vi "LvIRKit_ManageIRData.vi"(7 "filepath":path=path "C:/EISOL/LvIRKIt/samples/sample.dat", 8 "action":T2(ring)=enum."Get", 9 "irdata":string, 10 "name":string, 11 "id":i32) -> (1 "irdata out":T1, 2 "IRDATA[]":T1[](array[typedef]))   [LabVIEW 2014]
uses:
  LvIRKit_rsc_IRData_typedef.ctl
panel:
  out "size of IRDATA[]":i32
  in  "irdata":T1
  # "JSONstring"
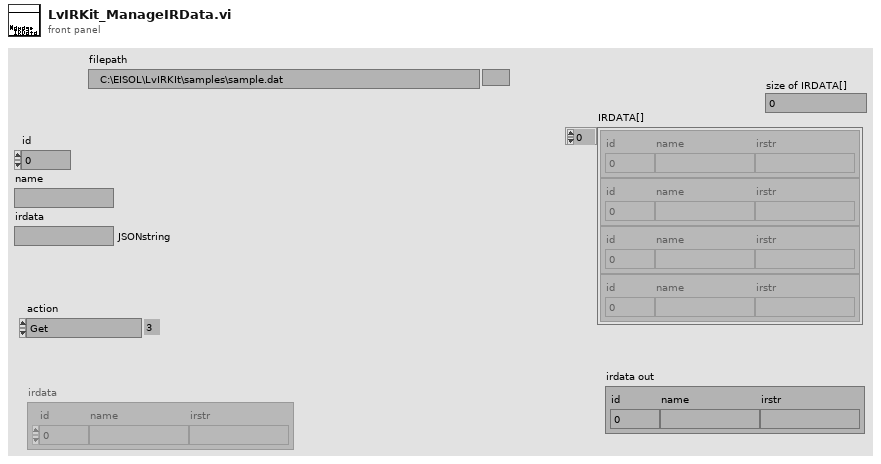
[diagram p1: front panel]
types:
  T1 = typedef "LvIRKit_rsc_IRData_typedef.ctl" = cluster{"id":i32, "name":string, "irstr":string}
  T2 = enum16{"Init", "Load", "Save", "Get", "Add", "Remove", "Replace", "Up", "Down"}
  T3 = enum16{"open", "replace", "create", "open or create", "replace or create", "replace or create with confirmation"}
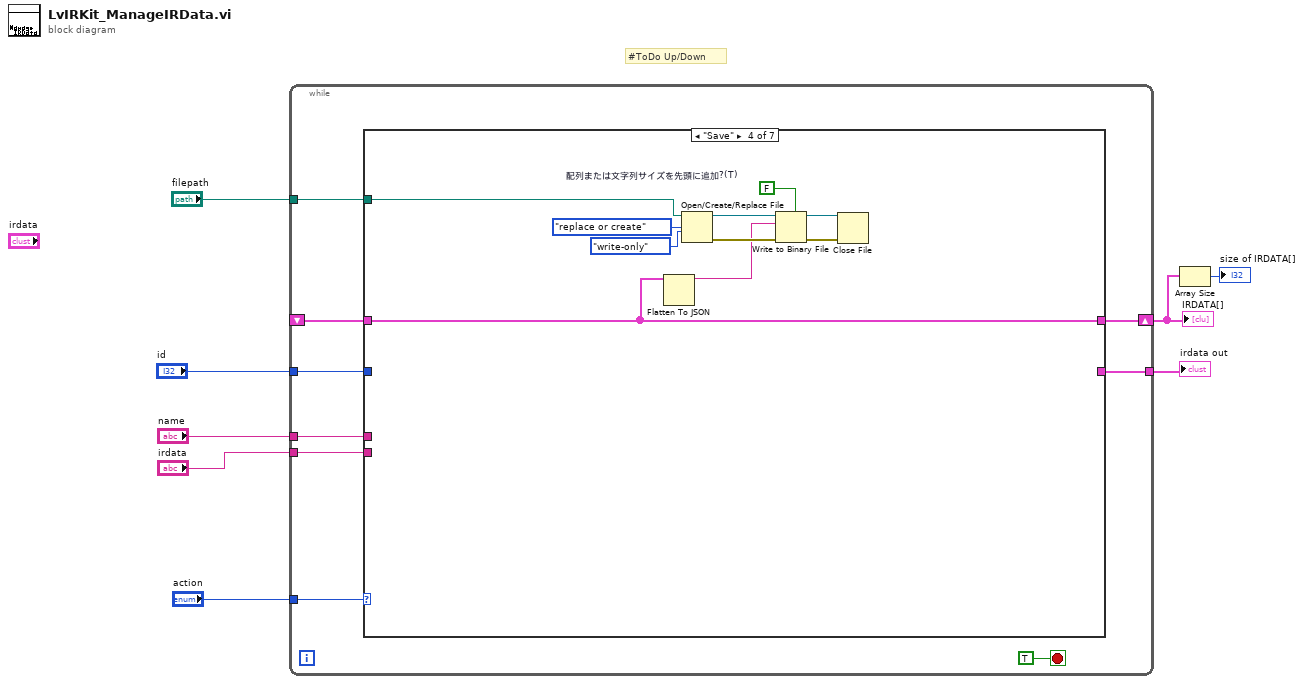
[diagram p0: block diagram]
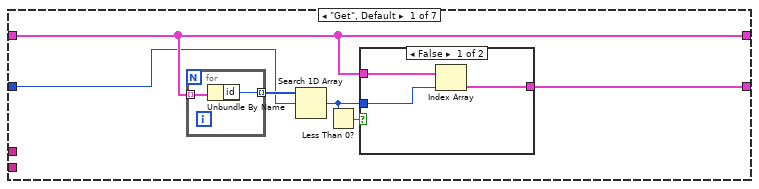
[diagram p2: hidden frame]
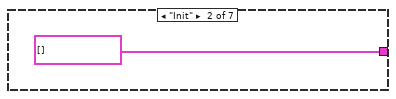
[diagram p4: hidden frame]
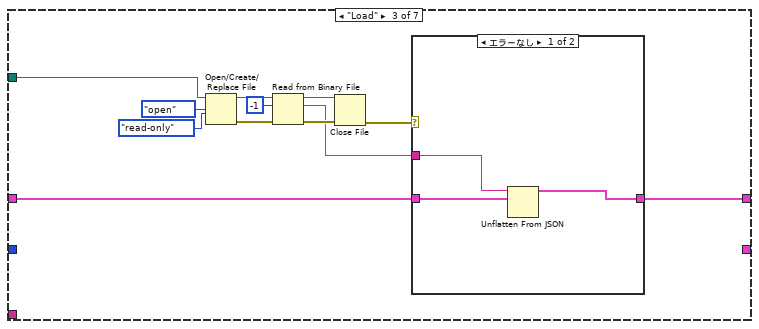
[diagram p5: hidden frame]
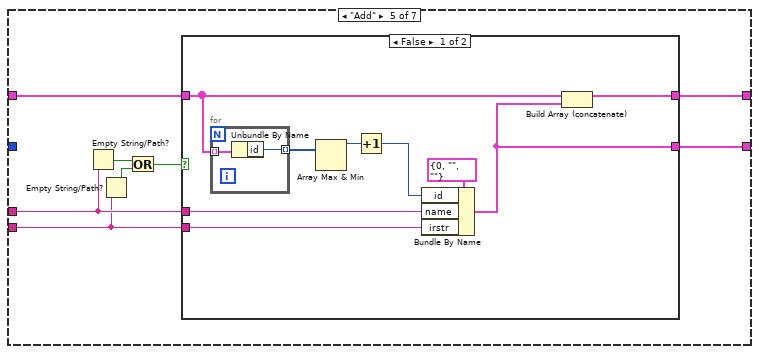
[diagram p7: hidden frame]
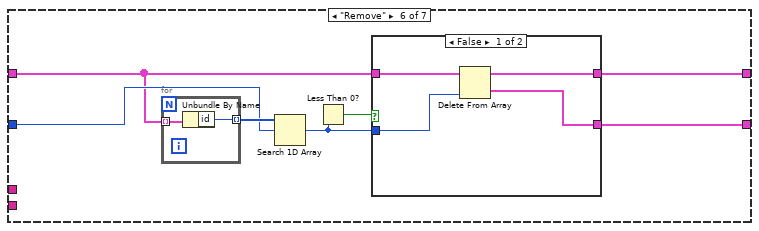
[diagram p9: hidden frame]
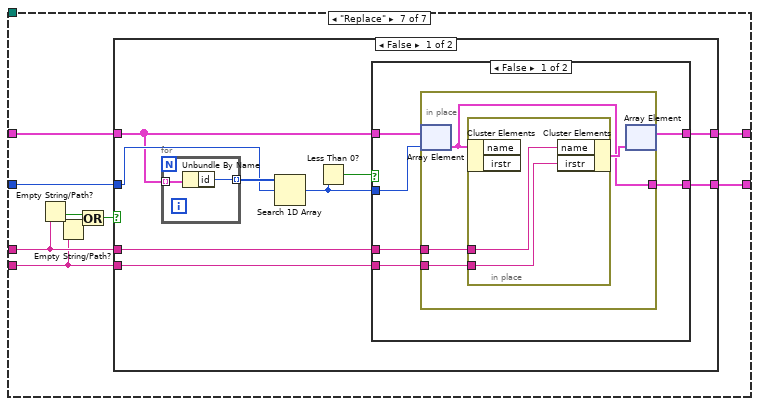
[diagram p11: hidden frame]
diagram:
  # "#ToDo Up/Down"
  n1 = while {
    tunnel: "action" -> [w16]
    shift-right: [w15] -> w2
    shift-left: _ -> [w14]
    tunnel: "id" -> [w13]
    tunnel: [w12] -> w6
    tunnel: "name" -> [w11]
    tunnel: "irdata" -> [w10]
    tunnel: "filepath" -> [w9]
    stop <- TRUE stop-if-true
    n2 = case shown="\"Save\"" w16 {
      tunnel: [w22 T1[] [] ("IRDATA[]") w32 w49 w63 w77 w96] -> w15
      tunnel: w14 -> [w22 _ w33 w49 w62 w78 w97]
      tunnel: w13 -> [w20 _ _ _ _ w81 w98]
      tunnel: [w23 _ _ _ w61 w76 w95] -> w12
      tunnel: w11 -> [_ _ _ _ w60 _ w94]
      tunnel: w10 -> [_ _ _ _ w59 _ w93]
      tunnel: w9 -> [_ _ w31 w46 _ _ _]
      frame "Get", Default {
        n3 = for {
          tunnel: w22 -> [w28] mode=indexing
          tunnel: [w27] -> w21 mode=indexing
          n4 = Unbundle By Name(w28) -> ("id"=w27:i32)
        }
        n5 = Search 1D Array(1D array=w21, element=w20) -> (index of element=w19:i32)  [unwired: 1 in]
        n6 = Less Than 0?(x=w19) -> (x < 0?=w18:bool)
        n7 = case shown="FALSE" w18 {
          tunnel: [w26 _] -> w23
          tunnel: w22 -> [w25 _]
          tunnel: w19 -> [w24 _]
          frame False {
            n8 = Index Array(array=w25, index=w24) -> (element=w26:T1)
          }
          frame True {
          }
        }
      }
      frame "Init" {
      }
      frame "Load" {
        n9 = Open/Create/Replace File(file path (use dialog)=w31, operation (0:open)=T3."open" ("操作（0:open）"), access (0:read/write)=enum16{"read/write", "read-only", "write-only"}."read-only" ("アクセス （0:read/write）")) -> (refnum out=w41:refnum<file>, error out=w40:errorcluster)  [unwired: 3 in, 1 out]
        n10 = Read from Binary File(8:w40, 10:-1 ("カウント（1）"), 11:w41) -> (0:w36:errorcluster, 2:w34:string, 3:w37:refnum<file>)  [unwired: 3 in, 1 out]
        n11 = Close File(refnum=w37, error in=w36) -> (error out=w35:errorcluster)  [unwired: 1 out]
        n12 = case shown="エラーなし" w35 {
          tunnel: w34 -> [w43 _]
          tunnel: w33 -> [w44 w45]
          tunnel: [w42 w45] -> w32
          frame No Error {
            n13 = Unflatten From JSON(JSON string=w43, type and defaults=w44) -> (value=w42:T1[])  [unwired: 5 in, 1 out]
          }
          frame Error {
          }
        }
      }
      frame "Save" {
        w47 = FALSE  # 配列または文字列サイズを先頭に追加?(T)
        n14 = Flatten To JSON(anything=w49) -> (JSON string=w48:string)  [unwired: 2 in, 1 out]
        n15 = Open/Create/Replace File(file path (use dialog)=w46, operation (0:open)=T3."replace or create" ("操作（0:open）"), access (0:read/write)=enum16{"read/write", "read-only", "write-only"}."write-only" ("アクセス （0:read/write）")) -> (refnum out=w55:refnum<file>, error out=w54:errorcluster)  [unwired: 3 in, 1 out]
        n16 = Write to Binary File(file (use dialog)=w55, data=w48, error in=w54, 5:w47) -> (refnum out=w51:refnum<file>, error out=w50:errorcluster)  [unwired: 2 in, 1 out]
        n17 = Close File(refnum=w51, error in=w50) -> ()  [unwired: 2 out]
      }
      frame "Add" {
        n18 = Empty String/Path?(string/path=w60) -> (empty?=w58:bool)
        n19 = Empty String/Path?(string/path=w59) -> (empty?=w57:bool)
        n20 = Or(x=w58, y=w57) -> (x .or. y?=w56:bool)
        n21 = case shown="FALSE" w56 {
          tunnel: [w72 w75] -> w63
          tunnel: w60 -> [w70 _]
          tunnel: w59 -> [w69 _]
          tunnel: w62 -> [w68 w75]
          tunnel: [w64 _] -> w61
          frame False {
            n22 = for {
              tunnel: w68 -> [w74] mode=indexing
              tunnel: [w73] -> w67 mode=indexing
              n23 = Unbundle By Name(w74) -> ("id"=w73:i32)
            }
            n24 = Array Max & Min(array=w67) -> (max value=w66:i32)  [unwired: 3 out]
            n25 = Increment(x=w66) -> (x+1=w65:i32)
            n26 = Bundle By Name(cluster=T1 {"id"=0, "name"="", "irstr"=""} ("irdata"), "id"=w65, "name"=w70, "irstr"=w69) -> (w64:T1)
            n27 = Build Array (concatenate)(w68, w64) -> (w72:T1[])
          }
          frame True {
          }
        }
      }
      frame "Remove" {
        n28 = for {
          tunnel: w78 -> [w84] mode=indexing
          tunnel: [w83] -> w82 mode=indexing
          n29 = Unbundle By Name(w84) -> ("id"=w83:i32)
        }
        n30 = Search 1D Array(1D array=w82, element=w81) -> (index of element=w80:i32)  [unwired: 1 in]
        n31 = Less Than 0?(x=w80) -> (x < 0?=w79:bool)
        n32 = case shown="FALSE" w79 {
          tunnel: w80 -> [w86 _]
          tunnel: w78 -> [w88 w89]
          tunnel: [w87 w89] -> w77
          tunnel: [w85 _] -> w76
          frame False {
            n33 = Delete From Array(array=w88, index=w86) -> (deleted portion=w85:T1, array with subset deleted=w87:T1[])  [unwired: 1 in]
          }
          frame True {
          }
        }
      }
      frame "Replace" {
        n34 = Empty String/Path?(string/path=w94) -> (empty?=w92:bool)
        n35 = Empty String/Path?(string/path=w93) -> (empty?=w91:bool)
        n36 = Or(x=w92, y=w91) -> (x .or. y?=w90:bool)
        n37 = case shown="FALSE" w90 {
          tunnel: w98 -> [w106 _]
          tunnel: w97 -> [w103 w123]
          tunnel: [w102 w123] -> w96
          tunnel: [w101 _] -> w95
          tunnel: w94 -> [w100 _]
          tunnel: w93 -> [w99 _]
          frame False {
            n38 = for {
              tunnel: w103 -> [w109] mode=indexing
              tunnel: [w108] -> w107 mode=indexing
              n39 = Unbundle By Name(w109) -> ("id"=w108:i32)
            }
            n40 = Search 1D Array(1D array=w107, element=w106) -> (index of element=w105:i32)  [unwired: 1 in]
            n41 = Less Than 0?(x=w105) -> (x < 0?=w104:bool)
            n42 = case shown="FALSE" w104 {
              tunnel: w105 -> [w110 _]
              tunnel: w103 -> [w115 w122]
              tunnel: [w114 w122] -> w102
              tunnel: [w113 _] -> w101
              tunnel: w100 -> [w112 _]
              tunnel: w99 -> [w111 _]
              frame False {
                n43 = in-place {
                  in-place-border: [w116] -> w113
                  in-place-border: w112 -> [w118]
                  in-place-border: w111 -> [w117]
                  n44 = in-place-array #1(w115, w110) -> (w116:T1)
                  n45 = in-place {
                    in-place-border: w118 -> [w121]
                    in-place-border: w117 -> [w120]
                    n46 = in-place-cluster #2(w116) -> ()  [unwired: 2 out]
                    n47 = in-place-cluster #2("name"=w121, "irstr"=w120) -> (w119:T1)
                  }
                  n48 = in-place-array #1(w119) -> (w114:T1[])  [unwired: 1 out]
                }
              }
              frame True {
              }
            }
          }
          frame True {
          }
        }
      }
    }
  }
  "IRDATA[]" <- w2
  "irdata out" <- w6
  n49 = Array Size(array=w2) -> (size(s)=→"size of IRDATA[]":i32)
